vi "TwGetDoubleAttributeFromH5.vi"(2 "name":string, 3 "location":string, 4 "filename":string, 5 "error in (no error)":errorcluster) -> (0 "attribute":dbl format="%.2f", 1 "error out":errorcluster)   [LabVIEW 2009]
uses:
  TwH5Dll.dll
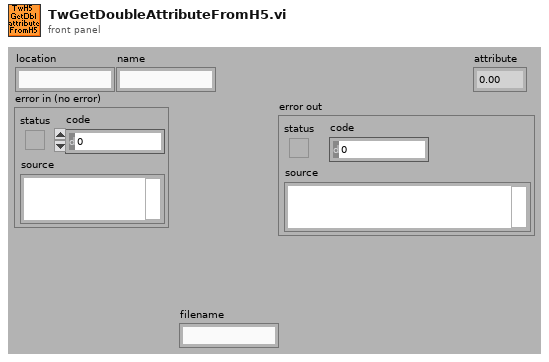
[diagram p1: front panel]
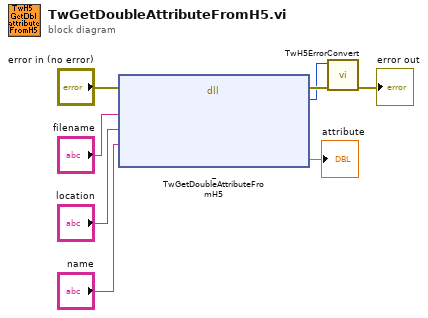
[diagram p0: block diagram]
diagram:
  n1 = dll-call lib="C:/src/85_TofDaq_current/DllWrappers/LabView/TwH5Dll/TwH5Dll.dll" fn="_TwGetDoubleAttributeFromH5"(error in="error in (no error)", "filename"="filename", "location"="location", "name"="name") -> (error out=w7:errorcluster, "TwRetVal"=w6:i32, "attribute"=→"attribute":dbl)  [unwired: 5 in, 2 out]
  n2 = call "TwH5ErrorConvert.vi"("error in (no error)"=w7, "error code"=w6) -> ("error out"=→"error out":errorcluster)  [unwired: 9 out]
